vi "Read Submodule EOL.vi"(8 "error in (no error)":errorcluster, 11 "Submodule EOL configuration":refnum<class "Submodule EOL configuration.lvclass">) -> (0 "error out":errorcluster, 2 "Submodule EOL":T1={"PLC Folder Names"=[], "Timeout Connect OPC"=0.0, "Connect OPC Trial"=0, "PLC URL"="", "Digitial IO"="", "HiPOT"="", "ACIR with Switch"="", "DMM with Switch"="", "Ignition Folder Names"=[], "Ignition URL"="", "Test Name"="Battery Submodule EOL"} {"Timeout Connect OPC" format="%#_f"}, 3 "Submodule EOL configuration out":refnum<class "Submodule EOL configuration.lvclass">)   [LabVIEW 2025, in "Submodule EOL.lvlib" / "Submodule EOL configuration.lvclass"]
uses:
  Submodule EOL configuration.lvclass
  Submodule EOL.ctl
  Submodule EOL configuration.lvclass/Submodule EOL configuration.ctl
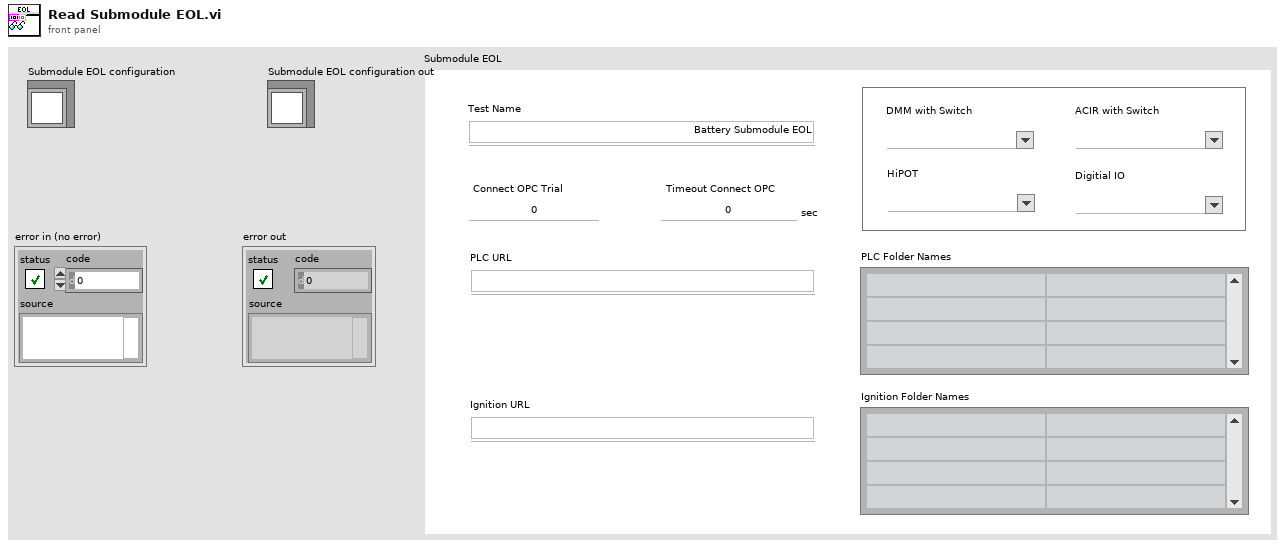
[diagram p1: front panel]
types:
  T1 = typedef "Submodule EOL.lvlib/Submodule EOL configuration.lvclass/Submodule EOL.ctl" = cluster{"PLC Folder Names":string[][], "Timeout Connect OPC":dbl, "Connect OPC Trial":u32, "PLC URL":string, "Digitial IO":string, "HiPOT":string, "ACIR with Switch":string, "DMM with Switch":string, "Ignition Folder Names":string[][], "Ignition URL":string, "Test Name":string}
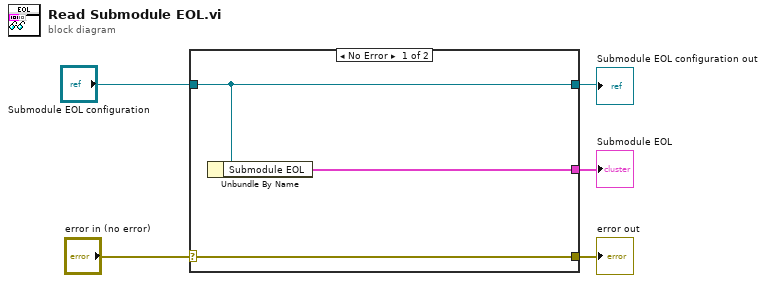
[diagram p0: block diagram]
diagram:
  n1 = case shown="No Error" "error in (no error)" {
    selector: "error in (no error)" -> [w8 w9]
    tunnel: [w8 w9] -> w4
    tunnel: [w7 w10] -> w2
    tunnel: "Submodule EOL configuration" -> [w7 w10]
    tunnel: [w6 _] -> w3
    frame No Error {
      n2 = Unbundle By Name(w7) -> ("Submodule EOL"=w6:T1)
    }
    frame Error {
    }
  }
  "error out" <- w4
  "Submodule EOL" <- w3
  "Submodule EOL configuration out" <- w2
